vi "Get SMO Public API.vi"(8 "error in (no error)":errorcluster, 11 "Example Instrument in":refnum<class "LevyLab Instrument.lvclass">) -> (0 "error out":errorcluster, 2 "Commands":string[](array[string]), 3 "Example Instrument out":refnum<class "LevyLab Instrument.lvclass">)   [LabVIEW 2019, in "LevyLab Instrument.lvclass"]
uses:
  LevyLab Instrument.lvclass
  SMOs/Instrument/Instrument.lvclass
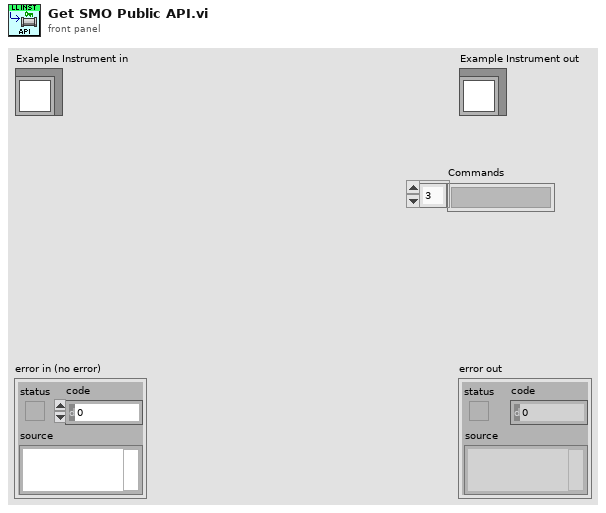
[diagram p1: front panel]
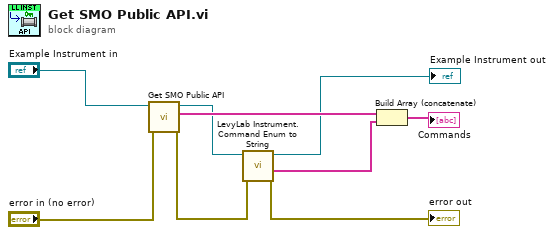
[diagram p0: block diagram]
diagram:
  n1 = call-parent "Get SMO Public API.vi"("error in (no error)"="error in (no error)", "Instrument in"="Example Instrument in") -> ("error out"=w5:errorcluster, "Commands"=w9:string[], "Instrument out"=w3:refnum<class "LevyLab Instrument.lvclass">)  [unwired: 7 in]
  n2 = call "LevyLab Instrument.Command Enum to String.vi"("error in (no error)"=w5, "LevyLab Instrument in"=w3) -> ("error out"=→"error out":errorcluster, "Commands []"=w1:string[], "LevyLab Instrument out"=→"Example Instrument out":refnum<class "LevyLab Instrument.lvclass">)  [unwired: 6 in, 1 out]
  n3 = Build Array (concatenate)(w9, w1) -> (→"Commands":string[])
